vi "PATCH Buffer.vi"(6 "timeout":i32=10000, 7 "output file":path, 8 "error in (no error)":errorcluster, 9 "buffer":string, 10 "url":string, 11 "HTTP Client Base in":refnum<class "LabVIEW HTTP Client.lvclass">) -> (0 "error out":errorcluster, 1 "body":string, 2 "headers":string, 3 "HTTP Client Base out":refnum<class "LabVIEW HTTP Client.lvclass">)   [LabVIEW 2020, in "HTTP Client Abstract.lvlib" / "LabVIEW HTTP Client.lvclass"]
uses:
  LabVIEW HTTP Client.lvclass
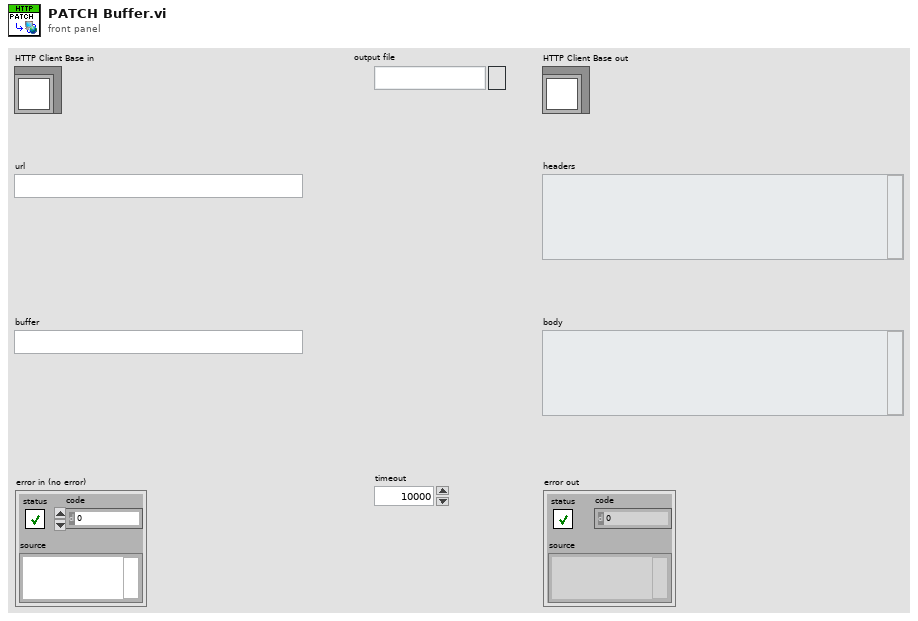
[diagram p1: front panel]
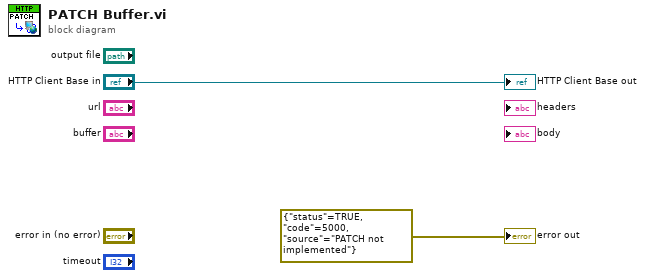
[diagram p0: block diagram]
diagram:
  "error out" <- errorcluster {"status"=TRUE, "code"=5000, "source"="PATCH not implemented"} ("error out")
  "HTTP Client Base out" <- "HTTP Client Base in"
